vi "DB Tools Load Recordset From File.vi"(4 "error in (no error)":errorcluster, 5 "cache size (1)":i32=1 min=1, 6 "file name":path, 7 "connection reference":T2) -> (0 "error out":errorcluster, 3 "recordset reference":T3)   [LabVIEW 2013, in "NI_Database_API_64.lvlib"]
doc: "Loads a recordset from a file and returns a <B>recordset reference</B> that identifies this recordset. You can retrieve data from this recordset like any other recordset, but some properties might not be available on this recordset."
uses:
  NI_Database_API_64.lvlib
  Connection.llb/Conn ObjectReference.ctl
  Rec ObjectReference.ctl
  Rec DataMembers.ctl
panel:
  in  "default":T1
  in  "default data":T1
  in  "ADODB._Recordset":refnum<k7>
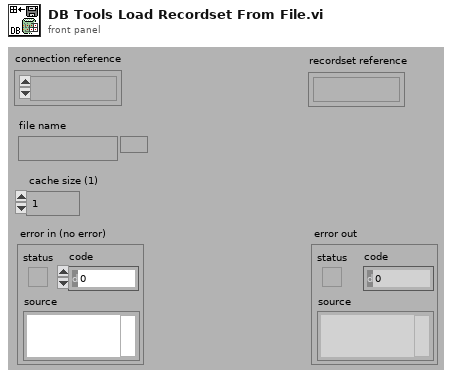
[diagram p1: front panel]
types:
  T1 = typedef "NI_Database_API_64.lvlib/Rec DataMembers.ctl" = cluster{"ADODB._Recordset":refnum<k7>, "Connection":T2}
  T2 = typedef "NI_Database_API_64.lvlib/Conn ObjectReference.ctl" = refnum<k1>
  T3 = typedef "NI_Database_API_64.lvlib/Rec ObjectReference.ctl" = refnum<k1>
  T4 = typedef "NI_Database_API_64.lvlib/Conn DataMembers.ctl" = cluster{"ADODB._Connection":refnum<k7>, "recordset objects":i32, "command objects":i32}
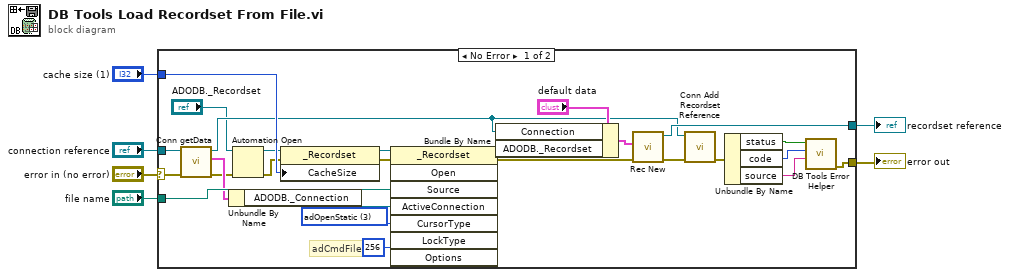
[diagram p0: block diagram]
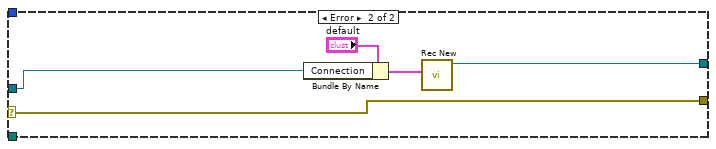
[diagram p2: hidden frame]
diagram:
  n1 = case shown="No Error" "error in (no error)" {
    selector: "error in (no error)" -> [w12 w37]
    tunnel: [w32 w33] -> w6
    tunnel: "cache size (1)" -> [w25 _]
    tunnel: "file name" -> [w21 _]
    tunnel: "connection reference" -> [w19 w34]
    tunnel: [w14 w37] -> w2
    frame No Error {
      w28 = 3 items=["adOpenUnspecified"=-1, "adOpenForwardOnly"=0, "adOpenKeyset"=1, "adOpenDynamic"=2, "adOpenStatic"=3] ("CursorType")
      # "adCmdFile"
      n2 = call "Conn getData.vi"("error in (no error)"=w12, "connection reference"=w19) -> ("error out"=w10:errorcluster, "data"=w20:T4, "connection reference out"=w18:T2)  [unwired: 3 out]
      n3 = Unbundle By Name(w20) -> ("ADODB._Connection"=w22:refnum<k7>)
      n4 = Automation Open(error in (no error)=w10, Automation Refnum="ADODB._Recordset") -> (Automation Refnum=w7:refnum<k7>, error out=w9:errorcluster)  [unwired: 2 out]
      n5 = property class="_Recordset"(reference=w7, error in=w9, "CacheSize"=w25) -> (reference out=w24:refnum<k7>, error out=w23:errorcluster)
      n6 = invoke class="_Recordset" method="Open"(reference=w24, error in=w23, "Source"=w21, "ActiveConnection"=w22, "CursorType"=w28, "Options"=256) -> (reference out=w30:refnum<k7>, error out=w29:errorcluster)  [unwired: 2 in, 6 out]
      n7 = Bundle By Name(cluster="default data", "Connection"=w18, "ADODB._Recordset"=w30) -> (w11:T1)
      n8 = call "Rec New.vi"("error in (no error)"=w29, "initial data"=w11) -> ("error out"=w26:errorcluster, "recordset reference"=w32:T3)  [unwired: 4 out]
      n9 = call "Conn Add Recordset Reference.vi"("error in (no error)"=w26, "connection reference"=w18) -> ("error out"=w15:errorcluster)  [unwired: 9 out]
      n10 = Unbundle By Name(w15) -> ("status"=w17:bool, "code"=w16:i32, "source"=w13:string)
      n11 = call "DB Tools Error Helper.vi"("source"=w13, "code"=w16, "status"=w17) -> ("error out"=w14:errorcluster)  [unwired: 1 in, 7 out]
    }
    frame Error {
      n12 = Bundle By Name(cluster="default", "Connection"=w34) -> (w35:T1)
      n13 = call "Rec New.vi"("initial data"=w35) -> ("recordset reference"=w33:T3)  [unwired: 1 in, 5 out]
    }
  }
  "recordset reference" <- w6
  "error out" <- w2
